vi "Configure Power On State.vi"(8 "error in (no error)":errorcluster, 10 "Output Power On Mode (0: Off)":i32(ring) items=["Off", "Auto", "On"], 11 "VISA resource name":refnum<visa-resource-name>) -> (0 "error out":errorcluster, 3 "VISA resource name out":refnum<visa-resource-name>)   [LabVIEW 2023]
doc: "Configures the output on/off setting at power-on."
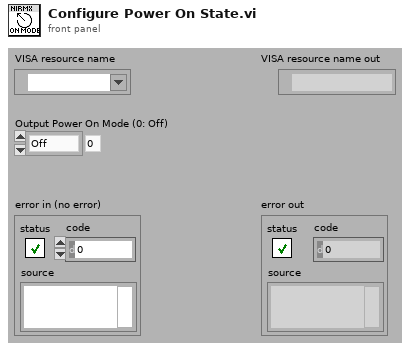
[diagram p1: front panel]
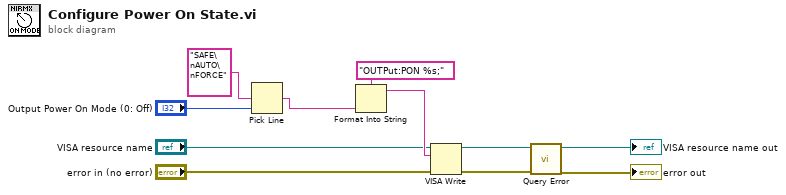
[diagram p0: block diagram]
diagram:
  n1 = Pick Line(multi-line string="SAFE\nAUTO\nFORCE" ("string (\"\")"), line index="Output Power On Mode (0: Off)") -> (output string=w2:string)  [unwired: 1 in]
  n2 = Format Into String(format string="OUTPut:PON %s;", w2) -> (resulting string=w10:string)  [unwired: 2 in, 1 out]
  n3 = VISA Write(VISA resource name="VISA resource name", write buffer=w10, error in (no error)="error in (no error)") -> (VISA resource name out=w7:refnum<visa-resource-name>, error out=w6:errorcluster)  [unwired: 1 out]
  n4 = call "Query Error.vi"("error in (no error)"=w6, "VISA resource name"=w7) -> ("error out"=→"error out":errorcluster, "VISA resource name out"=→"VISA resource name out":refnum<visa-resource-name>)  [unwired: 6 in, 2 out]
